vi "Unflatten LIDAR Data.vi"(8 "Odometry Data":dbl[](array[numeric]), 11 "LIDAR Data":cluster{"Magnitude":dbl[], "Direction":dbl[]}) -> (2 "Bearing (rad)":dbl[](array[numeric]), 3 "Range (m)":dbl[](array[numeric]))   [LabVIEW 2011]
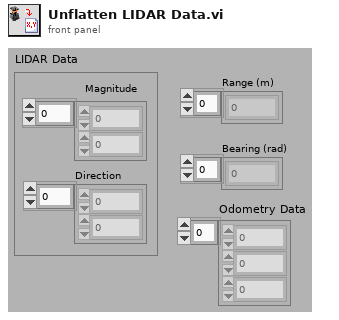
[diagram p1: front panel]
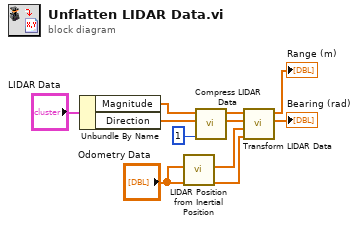
[diagram p0: block diagram]
diagram:
  n1 = Unbundle By Name("LIDAR Data") -> ("Magnitude"=w2:dbl[], "Direction"=w1:dbl[])
  n2 = call "LIDAR Position from Inertial Position.vi"("CM X, Y, Theta"="Odometry Data") -> ("LIDAR X, Y, Theta"=w6:dbl[])  [unwired: 10 in]
  n3 = call "Compress LIDAR Data.vi"("Compression Factor"=1 ("compress"), "Direction"=w1, "Magnitude"=w2) -> ("Compressed Direction"=w7:dbl[], "Compressed Magnitude"=w8:dbl[])  [unwired: 7 in]
  n4 = call "Transform LIDAR Data.vi"("New Orientation (X m, Y m, T rad)"="Odometry Data", "Orientation (X m, Y m, T rad)"=w6, "Direction (deg)"=w7, "Magnitude (mm)"=w8) -> ("Direction out (rad)"=→"Bearing (rad)":dbl[], "Magnitude out (m)"=→"Range (m)":dbl[])  [unwired: 5 in, 1 out]
